vi "Check And Create Folder.vi"(1 "Path In":path, 3 "String In":string) -> (0 "New Path out":path)   [LabVIEW 2024]
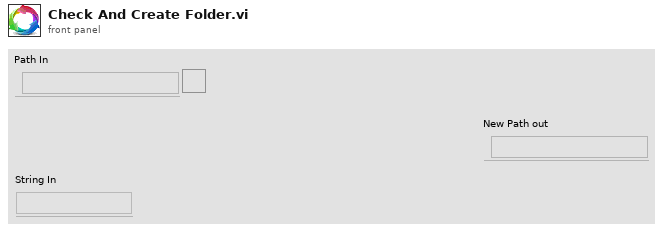
[diagram p1: front panel]
types:
  T1 = typedef "File Path Status.ctl" = enum16{"Path Doesn't Exist", "Path Exist", "Empty Path", "Not A Path"}
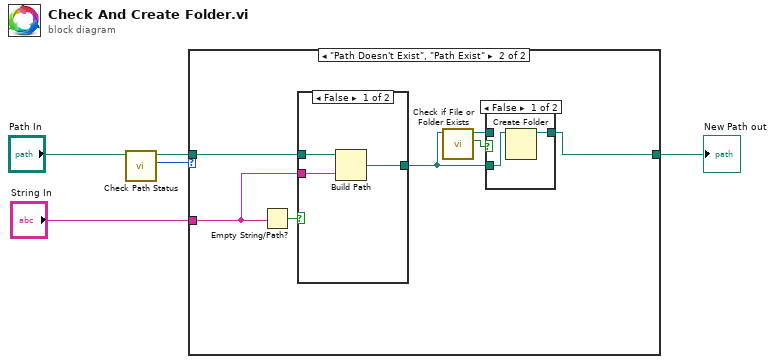
[diagram p0: block diagram]
diagram:
  n1 = call "Check Path Status.vi"("Path In"="Path In") -> ("File Path Status"=w1:T1, "Path Out"=w2:path)  [unwired: 9 in]
  n2 = case shown="\"Path Doesn't Exist\", \"Path Exist\"" w1 {
    tunnel: [w6 w10] -> w5
    tunnel: "String In" -> [_ w9]
    tunnel: w2 -> [w6 w7]
    frame "Empty Path", Default {
    }
    frame "Path Doesn't Exist", "Path Exist" {
      n3 = Empty String/Path?(string/path=w9) -> (empty?=w8:bool)
      n4 = case shown="False" w8 {
        tunnel: [w16 w17] -> w11
        tunnel: w7 -> [w15 w17]
        tunnel: w9 -> [w14 _]
        frame False {
          n5 = Build Path(base path=w15, name or relative path=w14) -> (appended path=w16:path)
        }
        frame True {
        }
      }
      n6 = call <vilib>:"Check if File or Folder Exists.vi"("path"=w11) -> ("file or folder exists?"=w13:bool, "dup path"=w12:path)  [unwired: 8 in, 1 out]
      n7 = case shown="False" w13 {
        tunnel: w12 -> [_ w20]
        tunnel: w11 -> [w19 _]
        tunnel: [w18 w20] -> w10
        frame False {
          n8 = Create Folder(path (use dialog)=w19) -> (created path=w18:path)  [unwired: 2 in, 2 out]
        }
        frame True {
        }
      }
    }
  }
  "New Path out" <- w5
